vi "Configuration Window.vi"(8 "error in (no error)":errorcluster, 11 "Instrument":refnum<class "Instrument.lvclass">) -> (0 "error out":errorcluster, 3 "Instrument out":refnum<class "Instrument.lvclass">)   [LabVIEW 2019, in "Instrument.lvlib" / "Instrument.lvclass"]
uses:
  Instrument.lvclass
  Instrument.lvclass/Instrument.ctl
panel:
  in  "Cancel":bool
  in  "Hardware Address":string
  in  "OK":bool
  # "Confirm or Make Changes:"
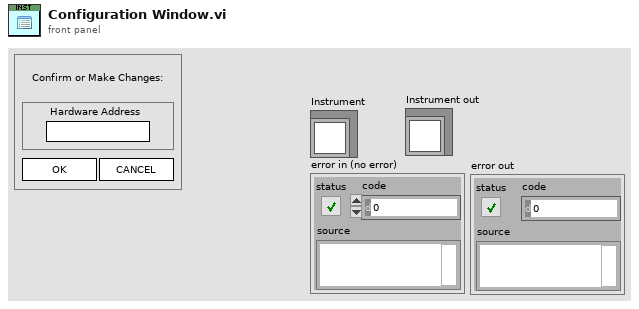
[diagram p1: front panel]
types:
  T1 = enum32{"Invalid", "Standard", "Closed", "Hidden", "Minimized", "Maximized"}
  T2 = enum32{"invalid app kind", "Development System", "Run Time System", "Student Edition", "Embedded LabVIEW", "Evaluation", "Custom"}
  T3 = typedef "Instrument.lvlib/Instrument.lvclass/Configuration--Cluster.ctl" = cluster{"Hardware":T4, "SMO":T5}
  T4 = typedef "Instrument.lvlib/Instrument.lvclass/HW Configuration--Cluster.ctl" = cluster{"address":string, "type":string}
  T5 = typedef "Instrument.lvlib/Instrument.lvclass/SMO Configuration--Cluster.ctl" = cluster{"Address":string, "Port":u16, "RC Type":T6, "Client Type":T7}
  T6 = typedef "RemoteControl.lvlib/RemoteControl.lvclass/RC Com Type--enum.ctl" = enum16{"RC", "STM", "ZMQ"}
  T7 = typedef "Instrument.lvlib/Instrument.lvclass/Client Type--Enum.ctl" = enum16{"Remote", "Local"}
  T8 = cluster{"Core":cluster{"Current VI Reference":refnum<vi>, "Close Panel on Exit?":bool}, "Configuration":T3}
  T9 = cluster{"Current VI Reference":refnum<vi>, "Close Panel on Exit?":bool}
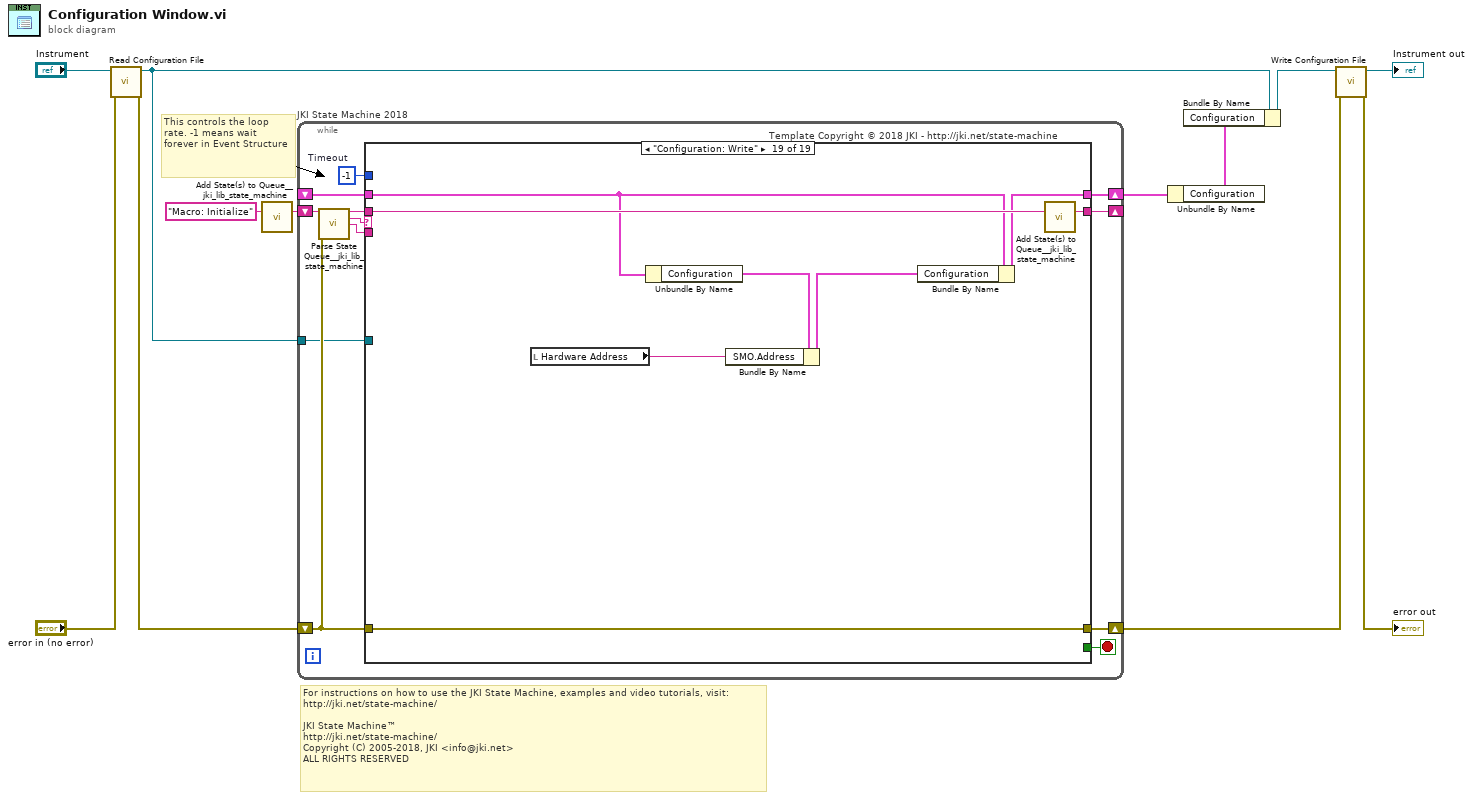
[diagram p0: block diagram]
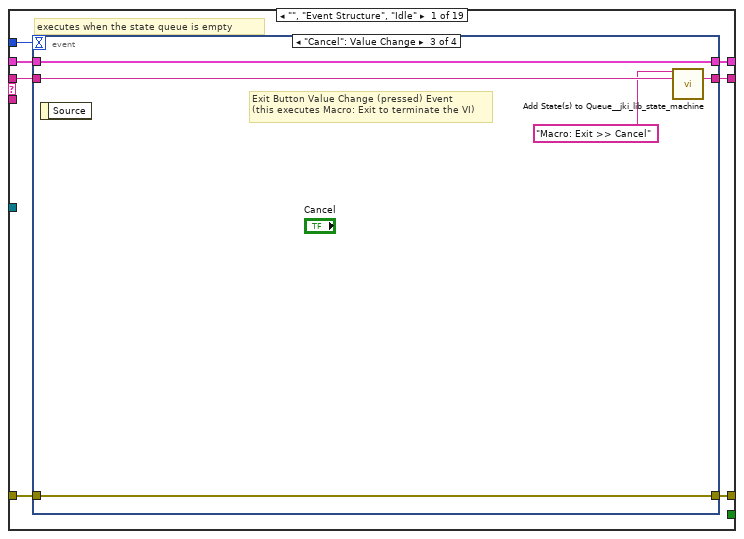
[diagram p2: hidden frame]
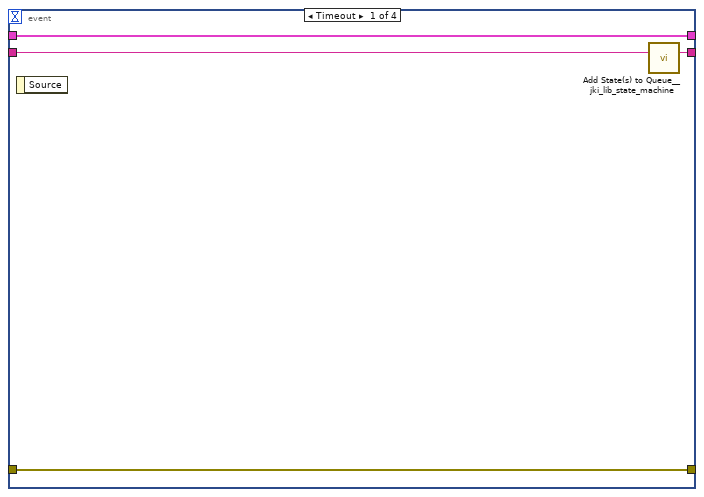
[diagram p3: hidden frame]
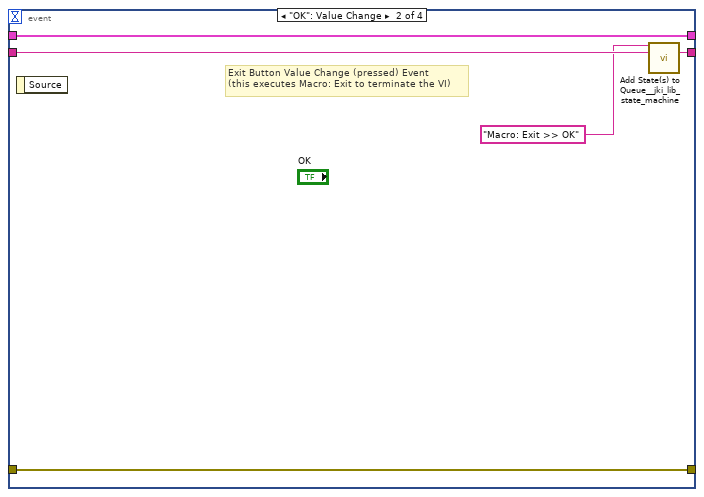
[diagram p4: hidden frame]
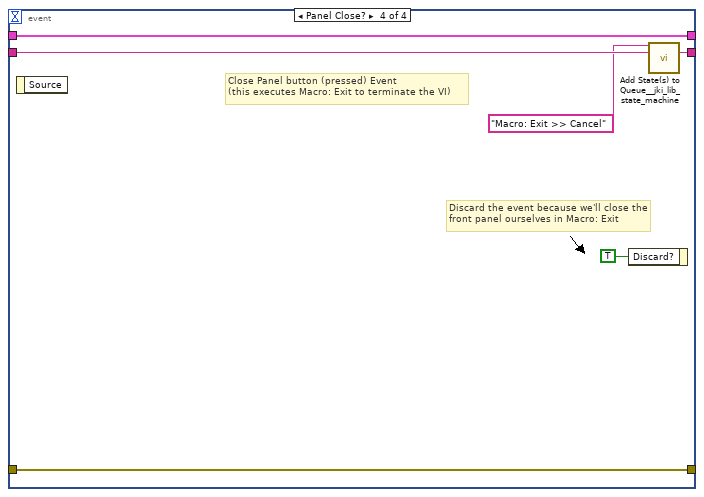
[diagram p5: hidden frame]
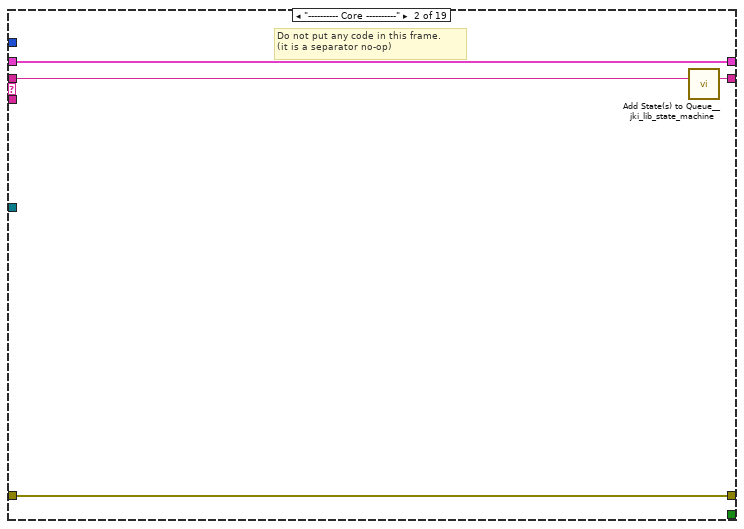
[diagram p6: hidden frame]
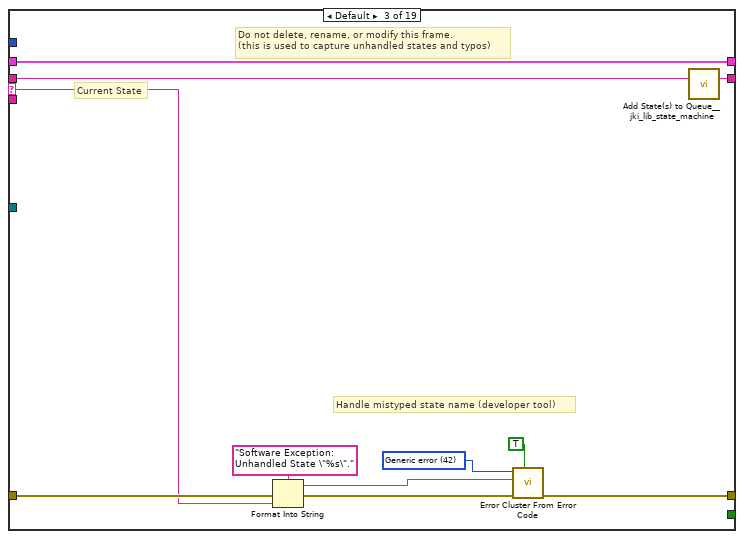
[diagram p7: hidden frame]
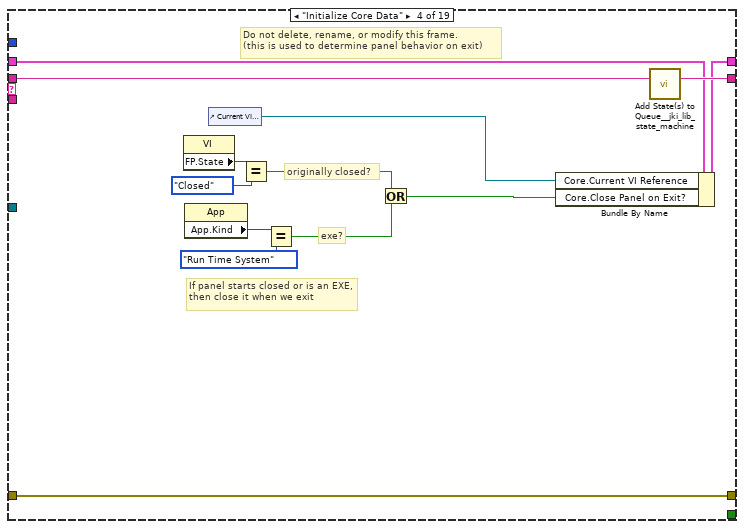
[diagram p8: hidden frame]
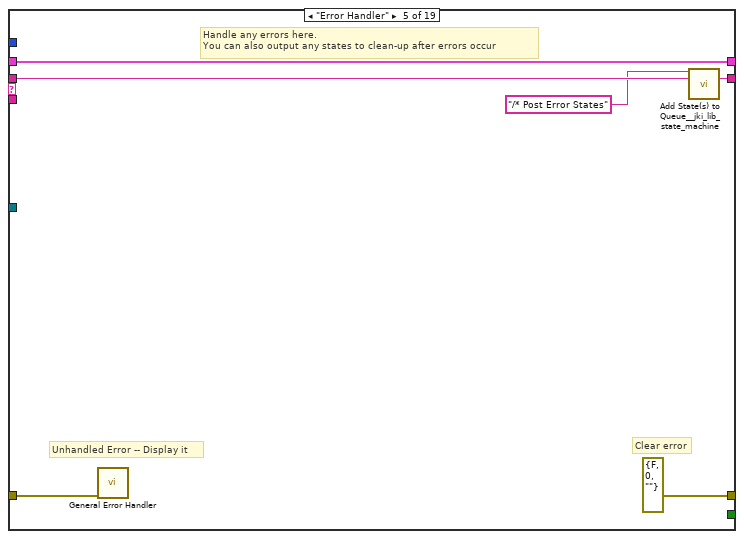
[diagram p9: hidden frame]
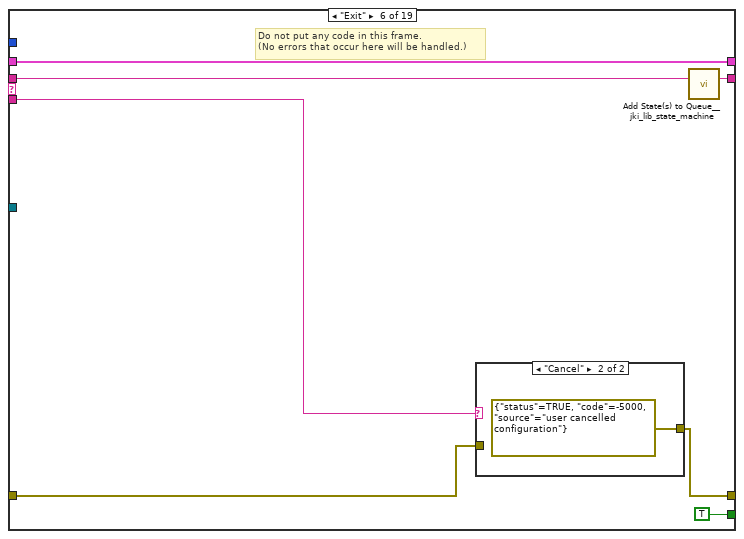
[diagram p10: hidden frame]
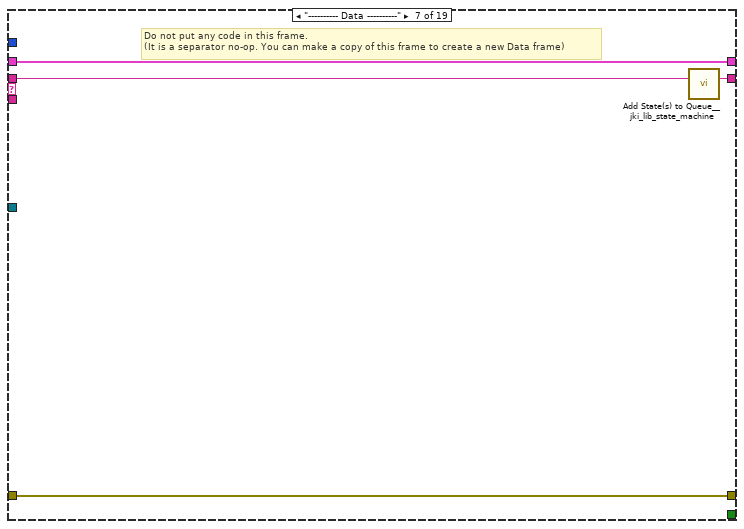
[diagram p12: hidden frame]
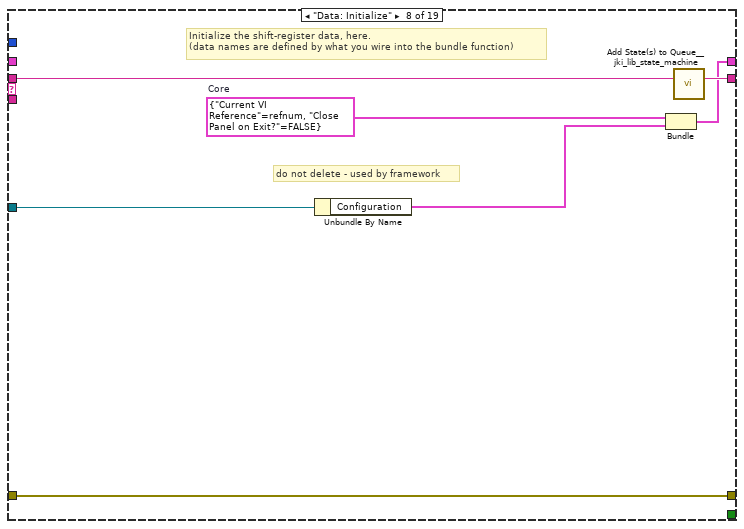
[diagram p13: hidden frame]
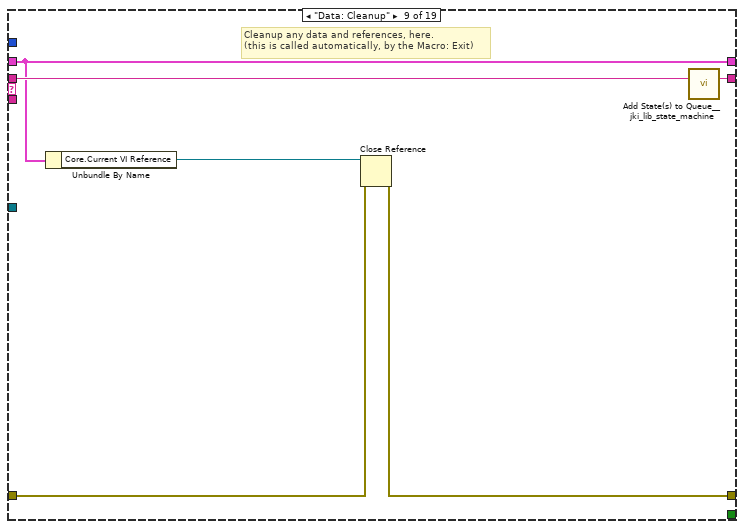
[diagram p14: hidden frame]
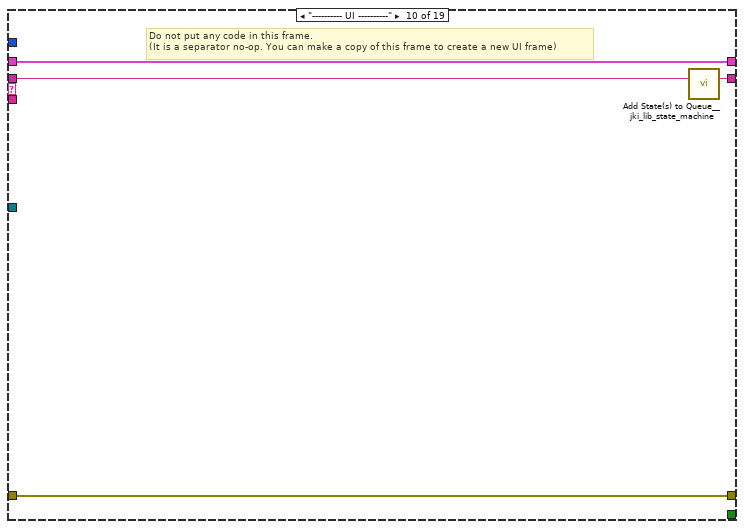
[diagram p15: hidden frame]
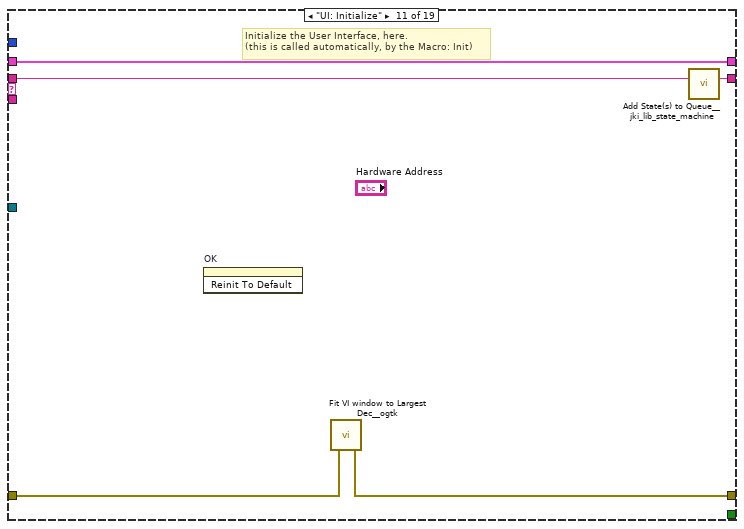
[diagram p16: hidden frame]
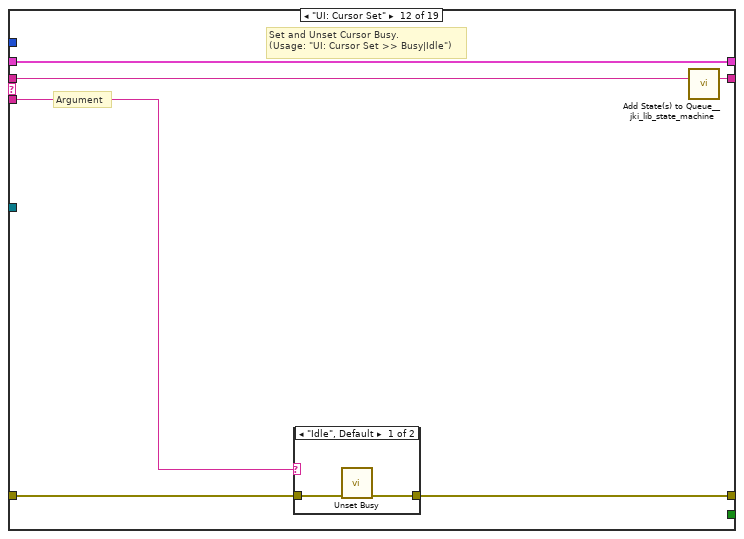
[diagram p17: hidden frame]
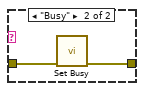
[diagram p18: hidden frame]
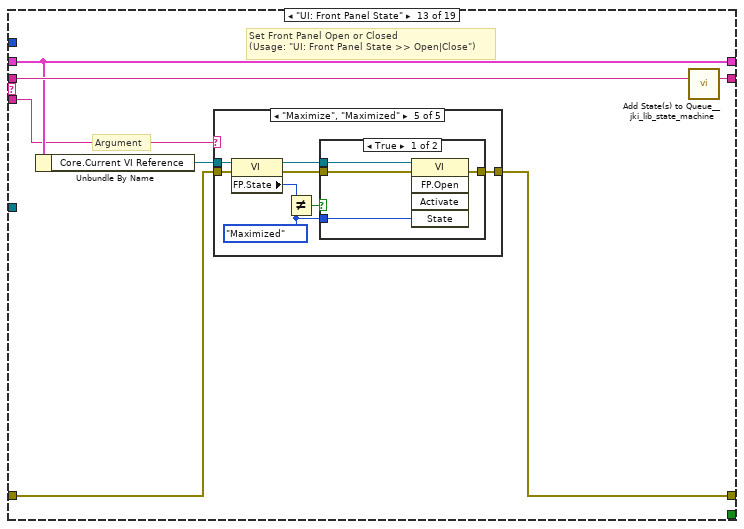
[diagram p19: hidden frame]
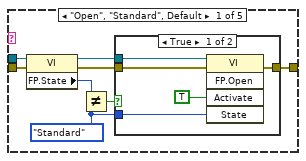
[diagram p20: hidden frame]
diagram:
  # "For instructions on how to use the JKI State Machine, examples and video tutorials, visit:\nhttp://jki.net/state-machine/\n\nJKI State Machine™\nhttp://jki.net/state-machine/\nCopyright (C) 2005-2018, JKI <info@jki.net>\nALL RIGHTS RESERVED"
  # "This controls the loop rate. -1 means wait forever in Event Structure"
  n1 = call-dynamic "Read Configuration File.vi"("error in (no error)"="error in (no error)", "Instrument in"="Instrument") -> ("error out"=w7:errorcluster, "Instrument out"=w2:refnum<class "Instrument.lvclass">)  [unwired: 8 in]
  n2 = call <vilib>:"Add State(s) to Queue__jki_lib_state_machine.vi"("State(s) in (\"\")"="Macro: Initialize") -> ("States Out"=w12:string)  [unwired: 14 in]
  n3 = while "JKI State Machine 2018" {
    shift-right: [w17] -> w10
    shift-left: _ -> [w16]
    shift-right: [w20] -> w4
    shift-left: w7 -> [w14]
    shift-right: [w19] -> _
    shift-left: w12 -> [w21]
    tunnel: w2 -> [w13]
    stop <- w18 stop-if-true
    w15 = -1  # Timeout
    # "Template Copyright © 2018 JKI - http://jki.net/state-machine"
    n4 = call <vilib>:"Parse State Queue__jki_lib_state_machine.vi"("State Queue"=w21, "Error In (no error)"=w14) -> ("Remaining States"=w23:string, "Current State"=w24:string, "Arguments"=w22:string)  [unwired: 11 in]
    n5 = case shown="\"Configuration: Write\"" w24 {
      selector: w24 -> [_ _ w56 _ _ _ _ _ _ _ _ _ _ _ _ _ _ _ _]
      tunnel: w23 -> [w31 w55 w60 w79 w85 w92 w98 w105 w111 w115 w120 w126 w137 w206 w211 w226 w230 w236 w244]
      tunnel: w22 -> [_ _ _ _ _ w88 _ _ _ _ _ w121 w131 _ _ w215 _ _ _]
      tunnel: w16 -> [w29 w52 w58 w72 w82 w90 w95 _ w106 w112 w118 w124 w133 w203 w208 w223 w227 w231 w240]
      tunnel: [w28 w53 w62 w76 errorcluster {"status"=FALSE, "code"=0, "source"=""} ("error out") w86 w96 w101 w107 w113 w116 w122 w134 w204 w209 w224 w228 w234 w237] -> w20
      tunnel: w14 -> [w27 w53 w61 w76 w81 w87 w96 w101 w108 w113 w117 w123 w135 w204 w209 w224 w228 w234 w237]
      tunnel: [w30 w54 w59 w78 w84 w91 w97 w104 w110 w114 w119 w125 w136 w205 w210 w225 w229 w235 w243] -> w19
      tunnel: [_ _ _ _ _ TRUE _ _ _ _ _ _ _ _ _ _ _ _ _] -> w18
      tunnel: [w26 w52 w58 w77 w82 w90 w95 w103 w106 w112 w118 w124 w133 w203 w208 w223 w227 w231 w239] -> w17
      tunnel: w15 -> [w25 _ _ _ _ _ _ _ _ _ _ _ _ _ _ _ _ _ _]
      tunnel: w13 -> [_ _ _ _ _ _ _ w99 _ _ _ _ _ _ _ _ _ _ _]
      frame "", "Event Structure", "Idle" {
        # "executes when the state queue is empty"
        n6 = event shown="[2] \"Cancel\": Value Change" {
          selector: _ -> [_ _ _ _]
          dyn-events: _ -> [_ _ _ _]
          timeout: w25 -> [_ _ _ _]
          tunnel: w31 -> [w35 w40 w45 w51]
          tunnel: [w34 w39 w44 w50] -> w30
          tunnel: w29 -> [w32 w37 w42 w48]
          tunnel: [w33 w38 w43 w49] -> w28
          tunnel: w27 -> [w33 w38 w43 w49]
          tunnel: [w32 w37 w42 w48] -> w26
          event Timeout {
            n7 = event-data() -> ()  [unwired: 1 in, 1 out]
            n8 = call <vilib>:"Add State(s) to Queue__jki_lib_state_machine.vi"("State(s) in (\"\")"=w35) -> ("States Out"=w34:string)  [unwired: 14 in]
          }
          event "OK": Value Change {
            # "Exit Button Value Change (pressed) Event\n(this executes Macro: Exit to terminate the VI)"
            n9 = event-data() -> ()  [unwired: 1 in, 1 out]
            n10 = call <vilib>:"Add State(s) to Queue__jki_lib_state_machine.vi"("State(s) in Front (\"\")"="Macro: Exit >> OK", "State(s) in (\"\")"=w40) -> ("States Out"=w39:string)  [unwired: 13 in]
          }
          event "Cancel": Value Change {
            # "Exit Button Value Change (pressed) Event\n(this executes Macro: Exit to terminate the VI)"
            n11 = event-data() -> ()  [unwired: 1 in, 1 out]
            n12 = call <vilib>:"Add State(s) to Queue__jki_lib_state_machine.vi"("State(s) in Front (\"\")"="Macro: Exit >> Cancel", "State(s) in (\"\")"=w45) -> ("States Out"=w44:string)  [unwired: 13 in]
          }
          event Panel Close? {
            # "Discard the event because we'll close the front panel ourselves in Macro: Exit"
            # "Close Panel button (pressed) Event\n(this executes Macro: Exit to terminate the VI)"
            n13 = event-data() -> ()  [unwired: 1 in, 1 out]
            n14 = event-data("Discard?"=TRUE) -> ()  [unwired: 1 in, 1 out]
            n15 = call <vilib>:"Add State(s) to Queue__jki_lib_state_machine.vi"("State(s) in Front (\"\")"="Macro: Exit >> Cancel", "State(s) in (\"\")"=w51) -> ("States Out"=w50:string)  [unwired: 13 in]
          }
        }
      }
      frame "---------- Core ----------" {
        # "Do not put any code in this frame.\n(it is a separator no-op)"
        n16 = call <vilib>:"Add State(s) to Queue__jki_lib_state_machine.vi"("State(s) in (\"\")"=w55) -> ("States Out"=w54:string)  [unwired: 14 in]
      }
      frame Default {
        w65 = 42 items=["No error", "Argument error", "Memory is full", "Out of zone", "End of file", "File already open", "Generic file I/O error", "File not found", "File permission error", "Disk is full", "Duplicate path", "Too many files open", "System feature not enabled", "Resource file not found", "Cannot add resource", "Resource not found", "Image not found", "Image memory error", "Pen does not exist", "Config type invalid", "Config token not found", "Config parse error", "Config memory error", "Bad external code format", "Bad external code offset", "External code not present", "Null window", "Destroy window error", "Null menu", "Print aborted", "Bad print record", "Print driver error", "Windows error during printing", "Memory error during printing", "Print dialog error", "Generic print error", "Invalid device refnum", "Device not found", "Device parameter error", "Device unit error", "Cannot open device", "Device call aborted", "Generic error", "Cancelled by user", "Object ID too low", "Object ID too high", "Object not in heap", "Unknown heap", "Unknown object (invalid DefProc)", "Unknown object (DefProc not in table)", "Message out of range", "Invalid (null) method", "Unknown message", "Manager call not supported", "Bad address", "Network operation in progress", "Network operation timed out", "Connection is busy", "Network attribute not supported", "Network error", "Address in use", "System out of memory", "Connection aborted", "Connection refused", "Not connected", "Already connected", "Connection closed", "Initialization error (interapplication manager)", "Bad occurrence", "Wait on unbound occurrence handler", "Occurrence queue overflow", "Datalog type conflict", "Unused", "Unrecognized type (interapplication manager)", "Memory corrupt", "Failed to make temporary DLL", "Old CIN version", "Drag socket not found", "Failed to load drop-object", "Failed to register OLE object", "Failed to release OLE object", "Format specifier type mismatch", "Unknown format specifier", "Too few format specifiers", "Too many format specifiers", "Scan failed", "Newer CIN version", "Error converting to variant", "Runtime menu error", "Password tampered", "Variant attribute not found", "Incompatible variant data type", "Event data is not available", "Event Store is not present", "Occurrence is not found", "Event Queue is not created", "Event info is not available", "Refnum passed is NULL", "Error retrieving Class GUID", "Error retrieving CoClass GUID", "Error retrieving TypeLib GUID.", "Bad built application magic bytes.", "Specific driver is different from the specific driver associated with the Logical Name.", "There is no session opened to the class driver.", "Max Error", "MAX - Error with config objects", "MAX - Error loading configuration", "MAX - Group not supported"]
        # "Current State"
        # "Do not delete, rename, or modify this frame.\n(this is used to capture unhandled states and typos)"
        # "Handle mistyped state name (developer tool)"
        n17 = Format Into String(format string="Software Exception: Unhandled State \"%s\"." ("message"), error in=w61, w56) -> (resulting string=w64:string, error out=w63:errorcluster)  [unwired: 1 in]
        n18 = call <vilib>:"Error Cluster From Error Code.vi"("show call chain? (False)"=TRUE, "error in (no error)"=w63, "error message (\"\")"=w64, "error code (0)"=w65) -> ("error out"=w62:errorcluster)  [unwired: 5 in]
        n19 = call <vilib>:"Add State(s) to Queue__jki_lib_state_machine.vi"("State(s) in (\"\")"=w60) -> ("States Out"=w59:string)  [unwired: 14 in]
      }
      frame "Initialize Core Data" {
        # "Do not delete, rename, or modify this frame.\n(this is used to determine panel behavior on exit)"
        # "originally closed?"
        # "exe?"
        # "If panel starts closed or is an EXE, then close it when we exit"
        n20 = property class="VI"() -> ("FP.State"=w69:T1)  [unwired: 2 in, 2 out]
        n21 = property class="App"() -> ("App.Kind"=w75:T2)  [unwired: 2 in, 2 out]
        n22 = control-ref of="Current VI Reference"() -> (w70:refnum<vi>)
        n23 = Equal?(x=w69, y=T1."Closed" ("Front Panel Window:State")) -> (x = y?=w67:bool)
        n24 = Equal?(x=w75, y=T2."Run Time System" ("Application:Kind")) -> (x = y?=w73:bool)
        n25 = Or(x=w67, y=w73) -> (x .or. y?=w71:bool)
        n26 = Bundle By Name(cluster=w72, "Core.Current VI Reference"=w70, "Core.Close Panel on Exit?"=w71) -> (w77:T8)
        n27 = call <vilib>:"Add State(s) to Queue__jki_lib_state_machine.vi"("State(s) in (\"\")"=w79) -> ("States Out"=w78:string)  [unwired: 14 in]
      }
      frame "Error Handler" {
        # "Unhandled Error -- Display it"
        # "Handle any errors here.\nYou can also output any states to clean-up after errors occur"
        # "Clear error"
        n28 = call <vilib>:"General Error Handler.vi"("error in (no error)"=w81) -> ()  [unwired: 10 in, 5 out]
        n29 = call <vilib>:"Add State(s) to Queue__jki_lib_state_machine.vi"("State(s) in Front (\"\")"="/* Post Error States", "State(s) in (\"\")"=w85) -> ("States Out"=w84:string)  [unwired: 13 in]
      }
      frame "Exit" {
        # "Do not put any code in this frame.\n(No errors that occur here will be handled.)"
        n30 = case shown="\"Cancel\"" w88 {
          tunnel: w87 -> [w93 _]
          tunnel: [w93 errorcluster {"status"=TRUE, "code"=-5000, "source"="user cancelled configuration"} ("error in (no error)")] -> w86
          frame "OK", Default {
          }
          frame "Cancel" {
          }
        }
        n31 = call <vilib>:"Add State(s) to Queue__jki_lib_state_machine.vi"("State(s) in (\"\")"=w92) -> ("States Out"=w91:string)  [unwired: 14 in]
      }
      frame "---------- Data ----------" {
        # "Do not put any code in this frame.\n(It is a separator no-op. You can make a copy of this frame to create a new Data frame)"
        n32 = call <vilib>:"Add State(s) to Queue__jki_lib_state_machine.vi"("State(s) in (\"\")"=w98) -> ("States Out"=w97:string)  [unwired: 14 in]
      }
      frame "Data: Initialize" {
        w102 = T9 {"Current VI Reference"=refnum, "Close Panel on Exit?"=FALSE}  # Core
        # "do not delete - used by framework"
        # "Initialize the shift-register data, here.\n(data names are defined by what you wire into the bundle function)"
        n33 = Unbundle By Name(w99) -> ("Configuration"=w100:T3)
        n34 = Bundle("Core"=w102, "Configuration"=w100) -> (w103:T8)  [unwired: 1 in]
        n35 = call <vilib>:"Add State(s) to Queue__jki_lib_state_machine.vi"("State(s) in (\"\")"=w105) -> ("States Out"=w104:string)  [unwired: 14 in]
      }
      frame "Data: Cleanup" {
        # "Cleanup any data and references, here.\n(this is called automatically, by the Macro: Exit)"
        n36 = Unbundle By Name(w106) -> ("Core.Current VI Reference"=w109:refnum<vi>)
        n37 = Close Reference(reference=w109, error in (no error)=w108) -> (error out=w107:errorcluster)
        n38 = call <vilib>:"Add State(s) to Queue__jki_lib_state_machine.vi"("State(s) in (\"\")"=w111) -> ("States Out"=w110:string)  [unwired: 14 in]
      }
      frame "---------- UI ----------" {
        # "Do not put any code in this frame.\n(It is a separator no-op. You can make a copy of this frame to create a new UI frame)"
        n39 = call <vilib>:"Add State(s) to Queue__jki_lib_state_machine.vi"("State(s) in (\"\")"=w115) -> ("States Out"=w114:string)  [unwired: 14 in]
      }
      frame "UI: Initialize" {
        # "Initialize the User Interface, here.\n(this is called automatically, by the Macro: Init)"
        n40 = invoke on="OK" class="Bool" method="Reinit To Default"() -> ()  [unwired: 3 in, 3 out]
        n41 = call <userlib>:"Fit VI window to Largest Dec__ogtk.vi"("error in (no error)"=w117) -> ("error out"=w116:errorcluster)  [unwired: 5 in, 1 out]
        n42 = call <vilib>:"Add State(s) to Queue__jki_lib_state_machine.vi"("State(s) in (\"\")"=w120) -> ("States Out"=w119:string)  [unwired: 14 in]
      }
      frame "UI: Cursor Set" {
        # "Argument"
        # "Set and Unset Cursor Busy.\n(Usage: \"UI: Cursor Set >> Busy|Idle\")"
        n43 = case shown="\"Idle\", Default" w121 {
          tunnel: w123 -> [w128 w130]
          tunnel: [w127 w129] -> w122
          frame "Idle", Default {
            n44 = call <vilib>:"Unset Busy.vi"("error in (no error)"=w128) -> ("error out"=w127:errorcluster)  [unwired: 10 in]
          }
          frame "Busy" {
            n45 = call <vilib>:"Set Busy.vi"("error in (no error)"=w130) -> ("error out"=w129:errorcluster)  [unwired: 9 in, 1 out]
          }
        }
        n46 = call <vilib>:"Add State(s) to Queue__jki_lib_state_machine.vi"("State(s) in (\"\")"=w126) -> ("States Out"=w125:string)  [unwired: 14 in]
      }
      frame "UI: Front Panel State" {
        # "Argument"
        # "Set Front Panel Open or Closed\n(Usage: \"UI: Front Panel State >> Open|Close\")"
        n47 = Unbundle By Name(w133) -> ("Core.Current VI Reference"=w132:refnum<vi>)
        n48 = case shown="\"Maximize\", \"Maximized\"" w131 {
          tunnel: w135 -> [w143 w158 w169 w182 w195]
          tunnel: [w145 w159 w171 w184 w197] -> w134
          tunnel: w132 -> [w144 w156 w170 w183 w196]
          frame "Open", "Standard", Default {
            w138 = T1."Standard" ("State")
            n49 = property class="VI"(reference=w144, error in=w143) -> (reference out=w141:refnum<vi>, error out=w142:errorcluster, "FP.State"=w140:T1)
            n50 = Not Equal?(x=w140, y=w138) -> (x != y?=w139:bool)
            n51 = case shown="True" w139 {
              tunnel: [w149 w151] -> w145
              tunnel: w142 -> [w148 w151]
              tunnel: w141 -> [w147 _]
              tunnel: w138 -> [w146 _]
              frame True {
                n52 = invoke class="VI" method="FP.Open"(reference=w147, error in=w148, "Activate"=TRUE, "State"=w146) -> (error out=w149:errorcluster)  [unwired: 1 in, 4 out]
              }
              frame False {
              }
            }
          }
          frame "Close", "Closed" {
            n53 = property class="VI"(reference=w156, error in=w158) -> (reference out=w155:refnum<vi>, error out=w157:errorcluster, "FP.State"=w153:T1)
            n54 = Not Equal?(x=w153, y=T1."Closed" ("Front Panel Window:State")) -> (x != y?=w152:bool)
            n55 = case shown="True" w152 {
              tunnel: [w160 w163] -> w159
              tunnel: w157 -> [w160 w162]
              tunnel: w155 -> [_ w161]
              frame False {
              }
              frame True {
                n56 = invoke class="VI" method="FP.Close"(reference=w161, error in=w162) -> (error out=w163:errorcluster)  [unwired: 1 in, 2 out]
              }
            }
          }
          frame "Hidden", "Hide" {
            w164 = T1."Hidden" ("State")
            n57 = property class="VI"(reference=w170, error in=w169) -> (reference out=w167:refnum<vi>, error out=w168:errorcluster, "FP.State"=w166:T1)
            n58 = Not Equal?(x=w166, y=w164) -> (x != y?=w165:bool)
            n59 = case shown="True" w165 {
              tunnel: [w175 w176] -> w171
              tunnel: w168 -> [w174 w176]
              tunnel: w167 -> [w173 _]
              tunnel: w164 -> [w172 _]
              frame True {
                n60 = invoke class="VI" method="FP.Open"(reference=w173, error in=w174, "State"=w172) -> (error out=w175:errorcluster)  [unwired: 2 in, 4 out]
              }
              frame False {
              }
            }
          }
          frame "Minimize", "Minimized" {
            w177 = T1."Minimized" ("State")
            n61 = property class="VI"(reference=w183, error in=w182) -> (reference out=w180:refnum<vi>, error out=w181:errorcluster, "FP.State"=w179:T1)
            n62 = Not Equal?(x=w179, y=w177) -> (x != y?=w178:bool)
            n63 = case shown="True" w178 {
              tunnel: [w188 w189] -> w184
              tunnel: w181 -> [w187 w189]
              tunnel: w180 -> [w186 _]
              tunnel: w177 -> [w185 _]
              frame True {
                n64 = invoke class="VI" method="FP.Open"(reference=w186, error in=w187, "State"=w185) -> (error out=w188:errorcluster)  [unwired: 2 in, 4 out]
              }
              frame False {
              }
            }
          }
          frame "Maximize", "Maximized" {
            w190 = T1."Maximized" ("State")
            n65 = property class="VI"(reference=w196, error in=w195) -> (reference out=w193:refnum<vi>, error out=w194:errorcluster, "FP.State"=w192:T1)
            n66 = Not Equal?(x=w192, y=w190) -> (x != y?=w191:bool)
            n67 = case shown="True" w191 {
              tunnel: [w201 w202] -> w197
              tunnel: w194 -> [w200 w202]
              tunnel: w193 -> [w199 _]
              tunnel: w190 -> [w198 _]
              frame True {
                n68 = invoke class="VI" method="FP.Open"(reference=w199, error in=w200, "State"=w198) -> (error out=w201:errorcluster)  [unwired: 2 in, 4 out]
              }
              frame False {
              }
            }
          }
        }
        n69 = call <vilib>:"Add State(s) to Queue__jki_lib_state_machine.vi"("State(s) in (\"\")"=w137) -> ("States Out"=w136:string)  [unwired: 14 in]
      }
      frame "---------- Macro ----------" {
        # "Do not put any code in this frame.\n(It is a separator no-op. You can make a copy of this frame to create a new Macro frame)"
        n70 = call <vilib>:"Add State(s) to Queue__jki_lib_state_machine.vi"("State(s) in (\"\")"=w206) -> ("States Out"=w205:string)  [unwired: 14 in]
      }
      frame "Macro: Initialize" {
        w207 = "Data: Initialize\nInitialize Core Data\nUI: Initialize\nUI: Front Panel State >> Open\nConfiguration: Read"  # Data: Initialize Initialize Core Data UI: Initialize UI: Front Panel State >> Open Configuration: Read
        # "Initialization Macro\n(This is called once, when the VI starts)"
        n71 = call <vilib>:"Add State(s) to Queue__jki_lib_state_machine.vi"("State(s) in Front (\"\")"=w207, "State(s) in (\"\")"=w211) -> ("States Out"=w210:string)  [unwired: 13 in]
      }
      frame "Macro: Exit" {
        # "Exit Macro\n(This is called once, when the VI exits)"
        n72 = Unbundle By Name(w223) -> ("Core.Close Panel on Exit?"=w222:bool)
        n73 = call <vilib>:"Build State String with Arguments__JKI_lib_State_Machine.vi"("Arguments (\"\")"=w215, "State"="Exit") -> ("State with Arguments"=w213:string)  [unwired: 4 in]
        n74 = Select(t="UI: Front Panel State >> Close", s=w222, f="") -> (s? t:f=w219:string)
        n75 = call <vilib>:"Add State(s) to Queue__jki_lib_state_machine.vi"("State(s) in Front (\"\")"="Data: Cleanup", "State(s) at Back (\"\")"=w213) -> ("States Out"=w212:string)  [unwired: 13 in]
        n76 = call <vilib>:"Add State(s) to Queue__jki_lib_state_machine.vi"("State(s) in Front (\"\")"="Configuration: Write", "State(s) in (\"\")"=w219, "State(s) at Back (\"\")"=w212) -> ("States Out"=w218:string)  [unwired: 12 in]
        n77 = call <vilib>:"Add State(s) to Queue__jki_lib_state_machine.vi"("State(s) in Front (\"\")"=w218, "State(s) in (\"\")"=w226) -> ("States Out"=w225:string)  [unwired: 13 in]
      }
      frame "---------- Configuration ----------" {
        # "Template Separator\n(You can make a copy of, or modify, this frame)"
        n78 = call <vilib>:"Add State(s) to Queue__jki_lib_state_machine.vi"("State(s) in (\"\")"=w230) -> ("States Out"=w229:string)  [unwired: 14 in]
      }
      frame "Configuration: Read" {
        # "Your code here.\n(You can make a copy of, or modify, this frame)"
        n79 = Unbundle By Name(w231) -> ("Configuration"=w232:T3)
        n80 = Unbundle By Name(w232) -> ("Hardware.address"=w233:string)  [unwired: 4 out]
        n81 = local write "Hardware Address"(w233) -> ()
        n82 = call <vilib>:"Add State(s) to Queue__jki_lib_state_machine.vi"("State(s) in (\"\")"=w236) -> ("States Out"=w235:string)  [unwired: 14 in]
      }
      frame "Configuration: Write" {
        n83 = local read "Hardware Address"() -> (w242:string)
        n84 = Unbundle By Name(w240) -> ("Configuration"=w241:T3)
        n85 = Bundle By Name(cluster=w241, "SMO.Address"=w242) -> (w238:T3)
        n86 = Bundle By Name(cluster=w240, "Configuration"=w238) -> (w239:T8)
        n87 = call <vilib>:"Add State(s) to Queue__jki_lib_state_machine.vi"("State(s) in (\"\")"=w244) -> ("States Out"=w243:string)  [unwired: 14 in]
      }
    }
  }
  n88 = Unbundle By Name(w10) -> ("Configuration"=w9:T3)
  n89 = Bundle By Name(cluster=w2, "Configuration"=w9) -> (w1:refnum<class "Instrument.lvclass">)
  n90 = call-dynamic "Write Configuration File.vi"("error in (no error)"=w4, "Instrument in"=w1) -> ("error out"=→"error out":errorcluster, "Instrument out"=→"Instrument out":refnum<class "Instrument.lvclass">)  [unwired: 8 in]
